vi "Window Chart.vi"(1 "error in":errorcluster, 2 "Display last":dbl[unit], 3 "Time per point (s)":dbl[unit], 4 "Waveform Chart":refnum<vi>) -> (0 "error out":errorcluster)   [LabVIEW 2009]
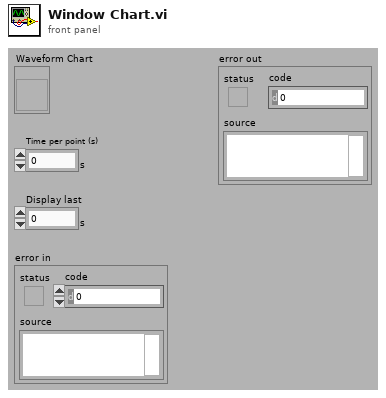
[diagram p1: front panel]
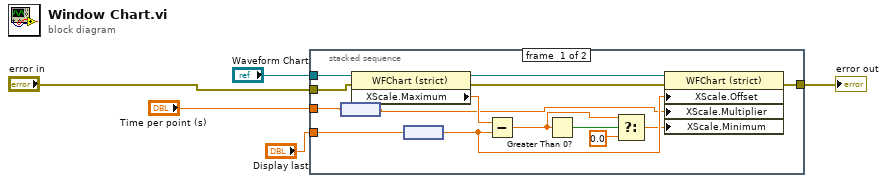
[diagram p0: block diagram]
diagram:
  n1 = stacked-sequence {
    tunnel: "Display last" -> [w11 _]
    tunnel: [w10 _] -> w5
    tunnel: "Waveform Chart" -> [w9 _]
    tunnel: "Time per point (s)" -> [w8 _]
    tunnel: "error in" -> [w6 _]
    frame #0 {
      n2 = node(w8) -> (w7:dbl)
      n3 = property on="Property Node" class="WFChart (strict)"(reference=w9, error in=w6) -> (reference out=w13:refnum<vi>, error out=w12:errorcluster, "XScale.Maximum"=w16:dbl)
      n4 = node(w11) -> (w15:dbl)
      n5 = Subtract(x=w16, y=w15) -> (x-y=w17:dbl)
      n6 = Greater Than 0?(x=w17) -> (x > 0?=w19:bool)
      n7 = Select(t=w17, s=w19, f=0.0) -> (s? t:f=w14:dbl)
      n8 = property on="Property Node" class="WFChart (strict)"(reference=w13, error in=w12, "XScale.Offset"=w15, "XScale.Multiplier"=w7, "XScale.Minimum"=w14) -> (error out=w10:errorcluster)  [unwired: 1 out]
    }
    frame #1 {
    }
  }
  "error out" <- w5
